vi "Demo_MakeDispBuff.vi"(1 "Channel":T1 items=["通道1", "通道2"], 2 "Type":enum16{"接收", "发送"}(ring)=enum."发送", 3 "OBJs":T2[](array[typedef])) -> (0 "Buffer":T3(array[cluster]) {"Channel" items=["通道1", "通道2"]})   [LabVIEW 2012]
uses:
  ControlCAN/ControlCAN.llb/VCI_CAN_OBJ.ctl
  ControlCAN/ControlCAN.llb/CAN Channel.ctl
  ControlCAN/ControlCAN.lvlib
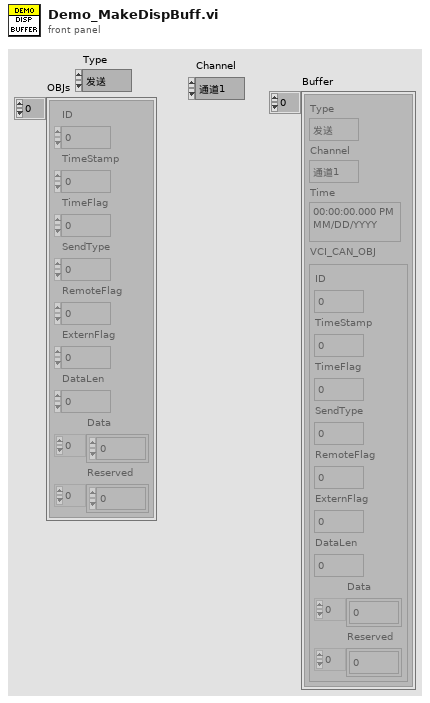
[diagram p1: front panel]
types:
  T1 = typedef "ControlCAN.lvlib/CAN Channel.ctl" = u32
  T2 = typedef "ControlCAN.lvlib/VCI_CAN_OBJ.ctl" = cluster{"ID":u32, "TimeStamp":u32, "TimeFlag":u8, "SendType":u8, "RemoteFlag":u8, "ExternFlag":u8, "DataLen":u8, "Data":u8[], "Reserved":u8[]}
  T3 = cluster{"Type":enum16{"接收", "发送"}, "Channel":T1, "Time":timestamp, "VCI_CAN_OBJ":T2}[]
  T4 = cluster{"Type":enum16{"接收", "发送"}, "Channel":T1, "Time":timestamp, "VCI_CAN_OBJ":T2}
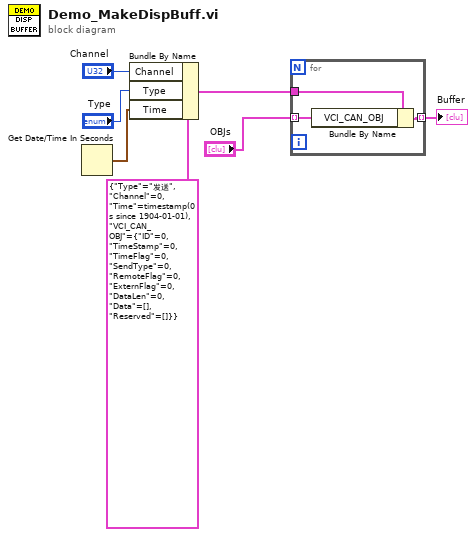
[diagram p0: block diagram]
diagram:
  n1 = Get Date/Time In Seconds() -> (seconds since 1Jan1904=w6:timestamp)
  n2 = Bundle By Name(cluster=T4 {"Type"=enum."发送", "Channel"=0, "Time"=timestamp(0 s since 1904-01-01), "VCI_CAN_OBJ"={"ID"=0, "TimeStamp"=0, "TimeFlag"=0, "SendType"=0, "RemoteFlag"=0, "ExternFlag"=0, "DataLen"=0, "Data"=[], "Reserved"=[]}}, "Channel"="Channel", "Type"="Type", "Time"=w6) -> (w5:T4)
  n3 = for {
    tunnel: w5 -> [w10]
    tunnel: [w9] -> w4 mode=indexing
    tunnel: "OBJs" -> [w8] mode=indexing
    n4 = Bundle By Name(cluster=w10, "VCI_CAN_OBJ"=w8) -> (w9:T4)
  }
  "Buffer" <- w4
